vi "Get Project Paths.vi"(8 "error in (no error)":errorcluster) -> (0 "error out":errorcluster, 1 "PlatformIO lib path":path, 2 "Firmware path":path, 3 "Repo Base":path)   [LabVIEW 2019, in "LINXx.lvlib"]
uses:
  LINXx.lvlib
panel:
  out "result":bool
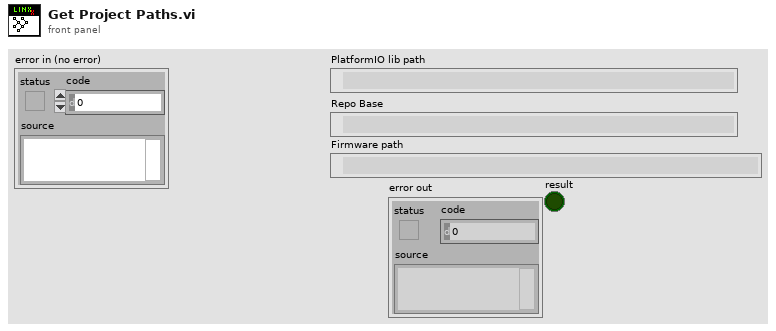
[diagram p1: front panel]
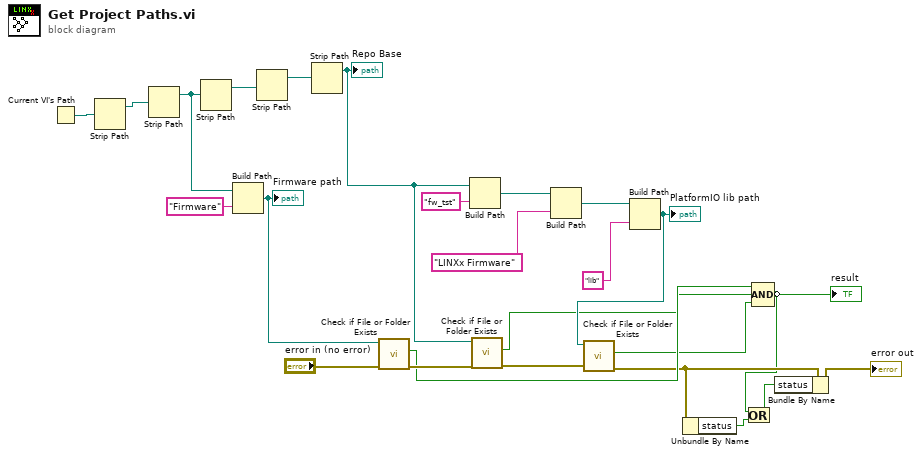
[diagram p0: block diagram]
diagram:
  n1 = Current VI's Path() -> (path=w25:path)
  n2 = Strip Path(path=w25) -> (stripped path=w24:path)  [unwired: 1 out]
  n3 = Strip Path(path=w24) -> (stripped path=w21:path)  [unwired: 1 out]
  n4 = Strip Path(path=w21) -> (stripped path=w23:path)  [unwired: 1 out]
  n5 = Build Path(base path=w21, name or relative path="Firmware") -> (appended path=w12:path)
  "Firmware path" <- w12
  n6 = Strip Path(path=w23) -> (stripped path=w22:path)  [unwired: 1 out]
  n7 = Strip Path(path=w22) -> (stripped path=w11:path)  [unwired: 1 out]
  "Repo Base" <- w11
  n8 = call <vilib>:"Check if File or Folder Exists.vi"("error in (no error)"="error in (no error)", "path"=w12) -> ("error out"=w14:errorcluster, "file or folder exists?"=w9:bool)  [unwired: 7 in, 1 out]
  n9 = Build Path(base path=w11, name or relative path="fw_tst") -> (appended path=w17:path)
  n10 = call <vilib>:"Check if File or Folder Exists.vi"("error in (no error)"=w14, "path"=w11) -> ("error out"=w13:errorcluster, "file or folder exists?"=w8:bool)  [unwired: 7 in, 1 out]
  n11 = Build Path(base path=w17, name or relative path="LINXx Firmware") -> (appended path=w16:path)
  n12 = Build Path(base path=w16, name or relative path="lib") -> (appended path=w10:path)
  "PlatformIO lib path" <- w10
  n13 = call <vilib>:"Check if File or Folder Exists.vi"("error in (no error)"=w13, "path"=w10) -> ("error out"=w4:errorcluster, "file or folder exists?"=w7:bool)  [unwired: 7 in, 1 out]
  n14 = Unbundle By Name(w4) -> ("status"=w3:bool)
  n15 = Compound Arithmetic op=AND(w9, w8, w7) -> (invert w2:bool)
  "result" <- w2
  n16 = Or(x=w2, y=w3) -> (x .or. y?=w1:bool)
  n17 = Bundle By Name(cluster=w4, "status"=w1) -> (→"error out":errorcluster)
